vi "Check for Discrete Input Mapping Conflicts.vi"(8 "error in (no error)":errorcluster, 11 "Coiil Group Ref in":T1 format="%.0x") -> (0 "error out":errorcluster, 1 "Conflicts?":bool, 2 "Conflicts":T2(array[cluster]), 3 "Coil Group Ref out":T1 format="%.0x")   [LabVIEW 2021, in "Modbus Master System Explorer.lvlib"]
uses:
  Modbus Master System Explorer.lvlib
  <vilib>/NI VeriStand/Custom Device API/Custom Device Item Ref.ctl
  SubVIs/Modbus Type.ctl
  <vilib>/NI VeriStand/Custom Device API/Custom Device API.lvlib
  Shared/Modbus Master Shared.lvlib
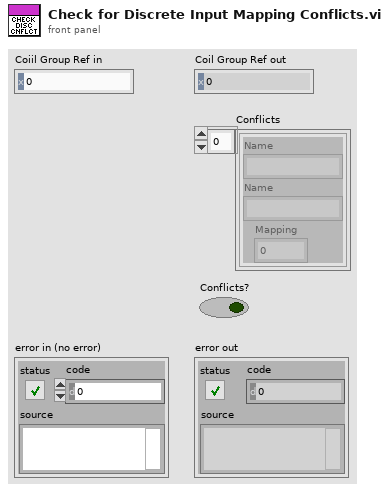
[diagram p1: front panel]
types:
  T1 = typedef "Custom Device API.lvlib/Custom Device Item Ref.ctl" = u64
  T2 = cluster{"Name":string, "Name":string, "Mapping":u16}[]
  T3 = typedef "Modbus Master Shared.lvlib/Modbus Type.ctl" = enum16{"Coil", "Discrete Input", "Holding Register", "Input Register"}
  T4 = typedef "Custom Device API.lvlib/Custom Device Item Info.ctl" = cluster{"Name":string, "Is Channel":bool, "GUID":string, "Is Waveform":bool}
  T5 = cluster{"Name":string, "Name":string, "Mapping":u16}
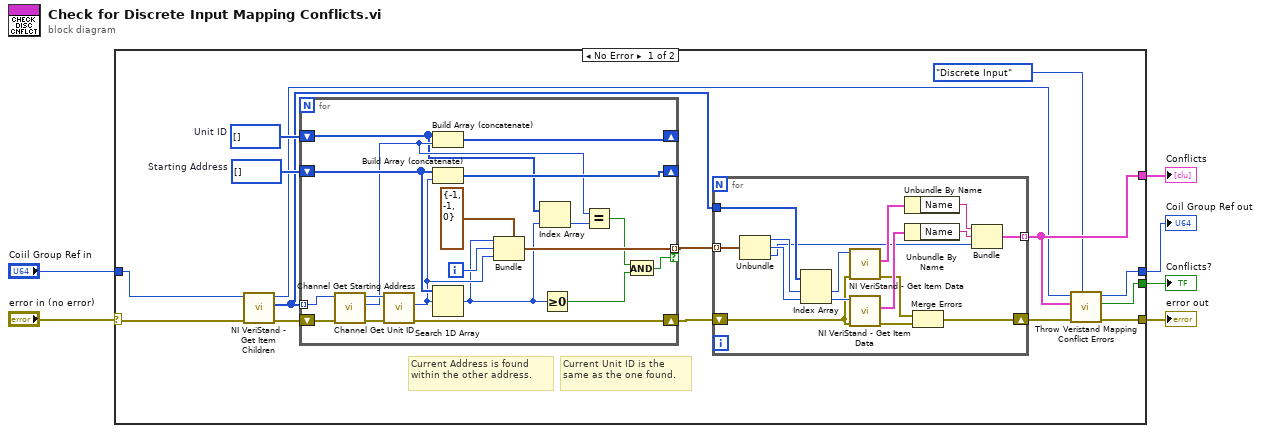
[diagram p0: block diagram]
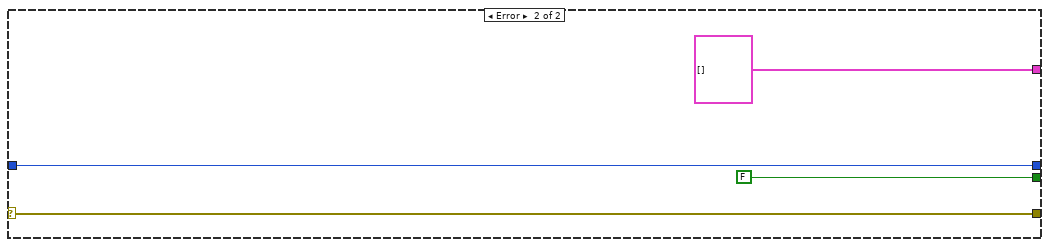
[diagram p2: hidden frame]
diagram:
  n1 = case shown="No Error" "error in (no error)" {
    selector: "error in (no error)" -> [w8 w58]
    tunnel: [w21 T2 []] -> w6
    tunnel: "Coiil Group Ref in" -> [w7 w59]
    tunnel: [w20 w58] -> w4
    tunnel: [w17 w59] -> w2
    tunnel: [w16 FALSE ("Conflicts?")] -> w1
    frame No Error {
      w13 = u8[] []  # Unit ID
      w15 = u16[] []  # Starting Address
      # "Current Unit ID is the same as the one found."
      # "Current Address is found within the other address."
      n2 = call <vilib>:"NI VeriStand - Get Item Children.vi"("error in (no error)"=w8, "Item Ref in"=w7) -> ("error out"=w14:errorcluster, "Child Refs"=w10:T1[], "Item Ref out"=w9:T1)  [unwired: 6 in, 1 out]
      n3 = for {
        tunnel: w10 -> [w46] mode=indexing
        shift-right: [w56] -> _
        shift-left: w15 -> [w55]
        tunnel: [w53] -> w11 mode=indexing if=w44
        shift-right: [w50] -> w12
        shift-left: w14 -> [w49]
        shift-right: [w43] -> _
        shift-left: w13 -> [w39]
        i -> [w52]
        n4 = call "Channel Get Unit ID.vi"("error in (no error)"=w49, "Item Ref in"=w46) -> ("error out"=w48:errorcluster, "Value"=w40:u8, "Item Ref out"=w47:T1)  [unwired: 7 in]
        n5 = call "Channel Get Starting Address.vi"("error in (no error)"=w48, "Item Ref in"=w47) -> ("error out"=w50:errorcluster, "Value"=w51:u16)  [unwired: 7 in, 1 out]
        n6 = Build Array (concatenate)(w39, w40) -> (w43:u8[])
        n7 = Build Array (concatenate)(w55, w51) -> (w56:u16[])
        n8 = Search 1D Array(1D array=w55, element=w51) -> (index of element=w42:i32)  [unwired: 1 in]
        n9 = Bundle(cluster=cluster{"y":i32, "y 2":i32, "Mapping":u16} {"y"=-1, "y 2"=-1, "Mapping"=0} ("Conflicting Indices"), "y"=w42, "y 2"=w52, "Mapping"=w51) -> (w53:cluster{"y":i32, "y 2":i32, "Mapping":u16})
        n10 = Index Array(array=w39, index=w42) -> (element=w41:u8)
        n11 = Greater Or Equal To 0?(x=w42) -> (x >= 0?=w45:bool)
        n12 = Equal?(x=w40, y=w41) -> (x = y?=w38:bool)
        n13 = And(x=w38, y=w45) -> (x .and. y?=w44:bool)
      }
      n14 = for {
        tunnel: w11 -> [w37] mode=indexing
        tunnel: w10 -> [w36]
        tunnel: [w27] -> w21 mode=indexing
        shift-right: [w22] -> w19
        shift-left: w12 -> [w25]
        n15 = Unbundle(w37) -> ("y"=w35:i32, "y 2"=w34:i32, "Mapping"=w26:u16)
        n16 = Index Array(array=w36, index #1=w35, index #2=w34) -> (element #1=w33:T1, element #2=w32:T1)
        n17 = call <vilib>:"NI VeriStand - Get Item Data.vi"("error in (no error)"=w25, "Item Ref in"=w33) -> ("error out"=w24:errorcluster, "Item Info"=w31:T4)  [unwired: 8 out]
        n18 = call <vilib>:"NI VeriStand - Get Item Data.vi"("error in (no error)"=w25, "Item Ref in"=w32) -> ("error out"=w23:errorcluster, "Item Info"=w30:T4)  [unwired: 8 out]
        n19 = Unbundle By Name(w31) -> ("Name"=w29:string)
        n20 = Unbundle By Name(w30) -> ("Name"=w28:string)
        n21 = Merge Errors(w24, w23) -> (w22:errorcluster)
        n22 = Bundle("Name"=w29, "Name"=w28, "Mapping"=w26) -> (w27:T5)  [unwired: 1 in]
      }
      n23 = call "Throw Veristand Mapping Conflict Errors.vi"("Type"=Modbus_Type."Discrete Input", "error in (no error)"=w19, "Conflicts In"=w21, "Item Ref in"=w9) -> ("error out"=w20:errorcluster, "Conflicts?"=w16:bool, "Node Ref out"=w17:T1)  [unwired: 5 in]
    }
    frame Error {
    }
  }
  "Conflicts?" <- w1
  "Conflicts" <- w6
  "Coil Group Ref out" <- w2
  "error out" <- w4
